vi "Launcher.vi"   [LabVIEW 2017]
uses:
  Controller/Controller/Controller.lvclass
  C:/Program Files (x86)/National Instruments/LabVIEW 2017/vi.lib/ActorFramework/Actor/Actor.lvclass
  <vilib>/ActorFramework/Actor/Actor.lvclass
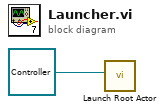
[diagram p0: block diagram]
diagram:
  n1 = call <vilib>:"Launch Root Actor.vi"("Actor"=refnum<class "Controller.lvclass"> refnum ("Error Handler.lvlib:Error Handler.lvclass")) -> ()  [unwired: 9 in, 2 out]
